vi "LIN_Data_Fold.vi"(10 "LIN Data array":T1[](array[typedef]) {"Properties" format="%x"}, 11 "Fold Data":bool) -> (2 "LIN Data array out":T1[](array[typedef]) {"Properties" format="%x"})   [LabVIEW 2014]
uses:
  Typedef/TLibLIN.ctl
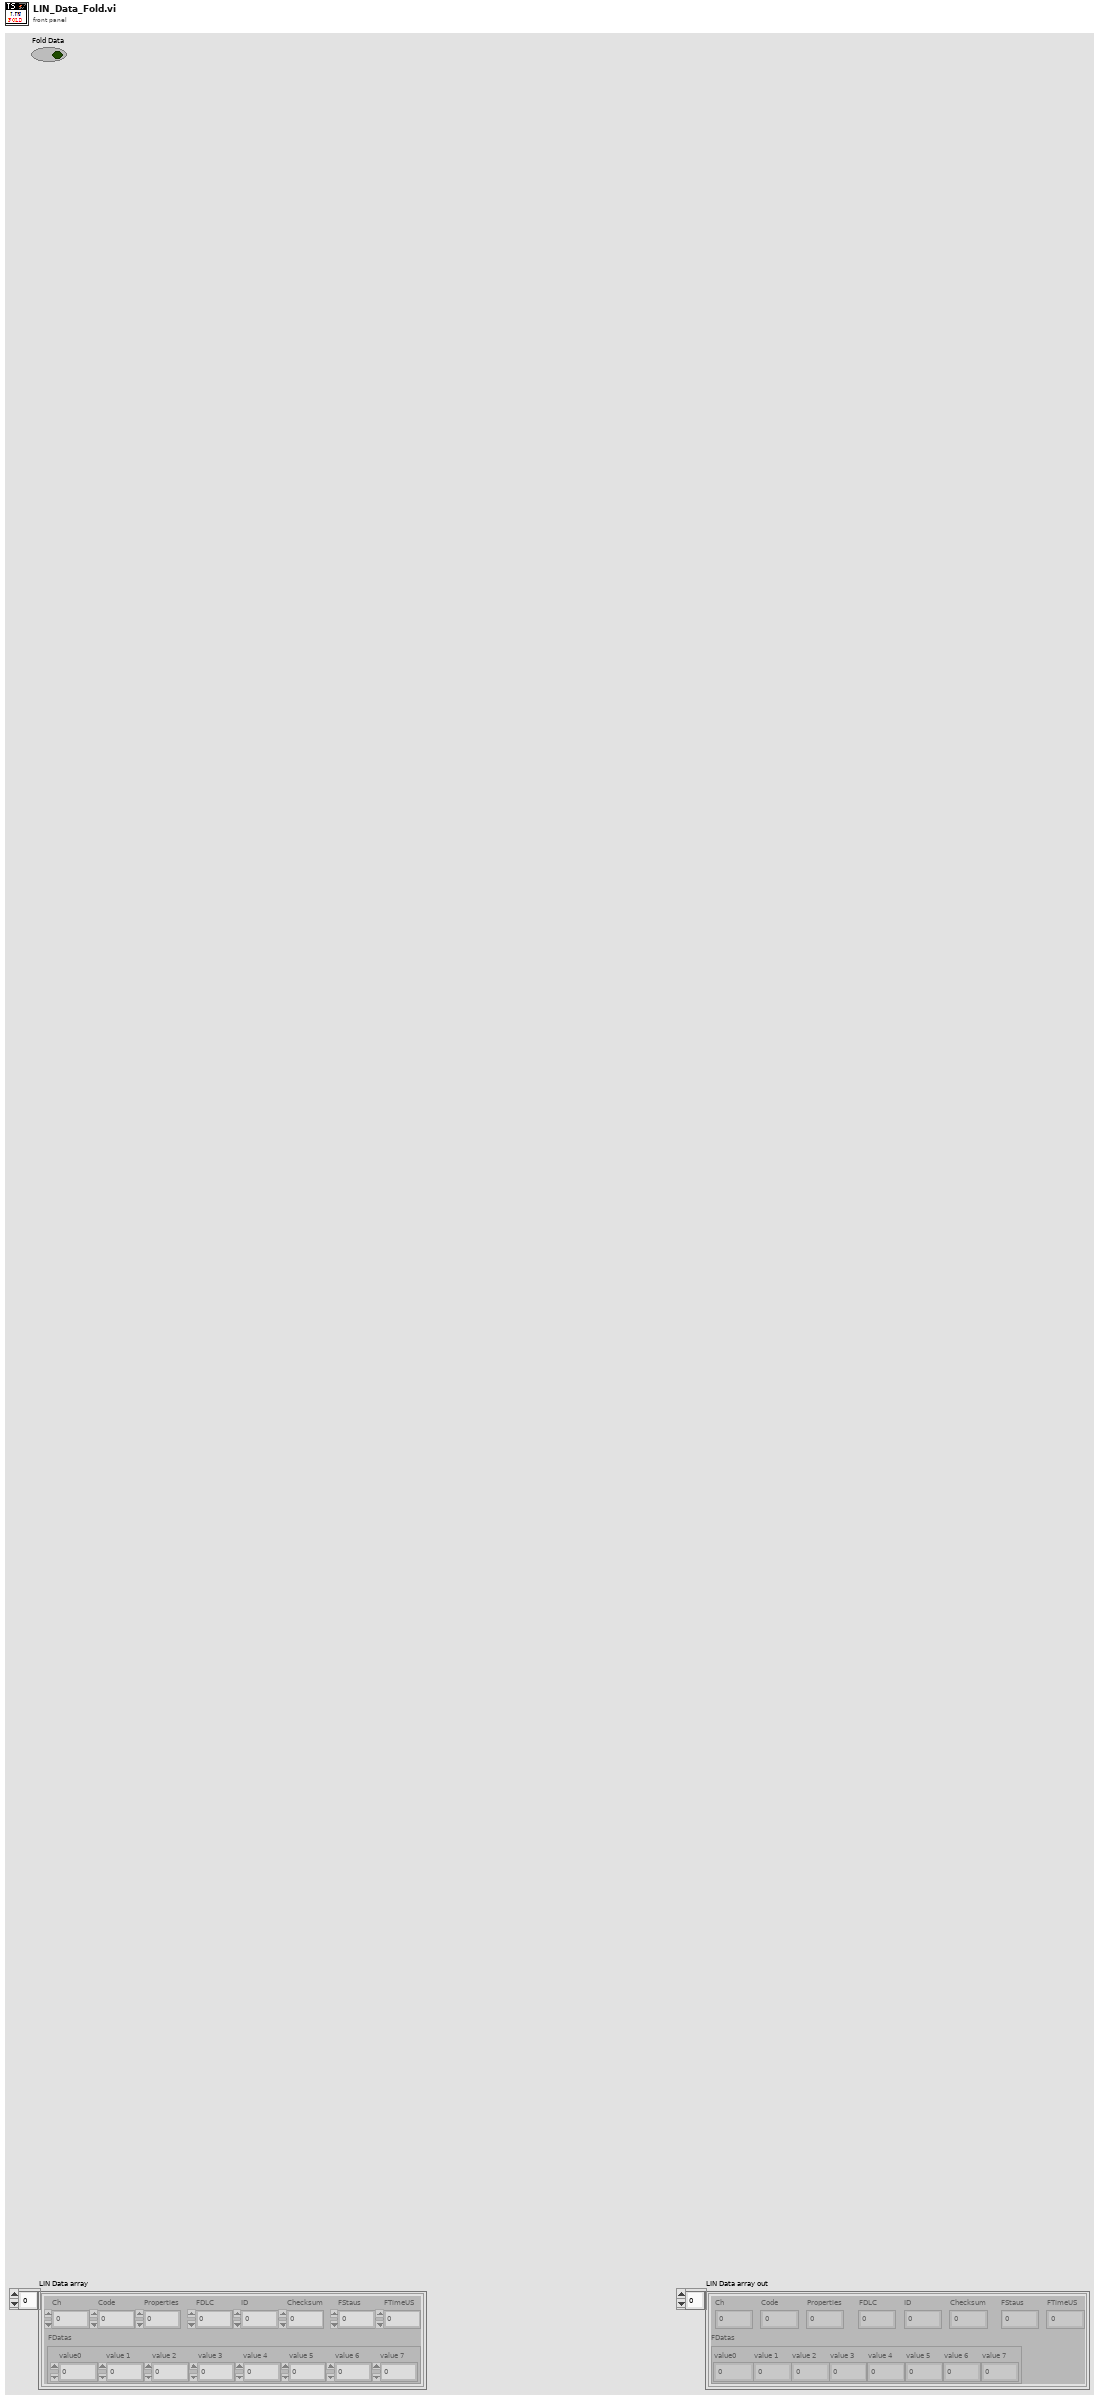
[diagram p1: front panel]
types:
  T1 = typedef "TLibLIN.ctl" = cluster{"Ch":u8, "Code":u8, "Properties":u8, "FDLC":u8, "ID":u8, "Checksum":u8, "FStaus":u8, "FTimeUS":u64, "FDatas":cluster{"value0":u8, "value 1":u8, "value 2":u8, "value 3":u8, "value 4":u8, "value 5":u8, "value 6":u8, "value 7":u8}}
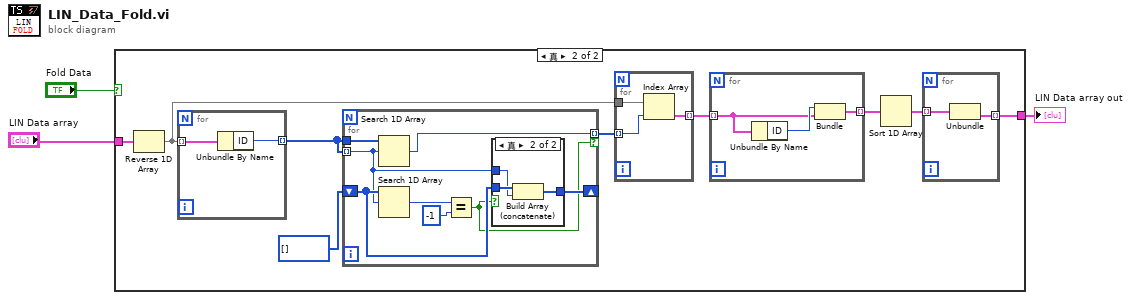
[diagram p0: block diagram]
diagram:
  n1 = case shown="真" "Fold Data" {
    tunnel: [w4 w12] -> w1
    tunnel: "LIN Data array" -> [w4 w6]
    frame False {
    }
    frame True {
      n2 = Reverse 1D Array(array=w6) -> (reversed array=w5:T1[])
      n3 = for {
        tunnel: w5 -> [w30] mode=indexing
        tunnel: [w29] -> w9 mode=indexing
        n4 = Unbundle By Name(w30) -> ("ID"=w29:u8)
      }
      n5 = for {
        tunnel: w9 -> [w19] mode=indexing
        shift-right: [w24] -> _
        shift-left: u32[] [] -> [w23]
        tunnel: [w18] -> w7 mode=indexing if=w17
        tunnel: w9 -> [w20]
        n6 = Search 1D Array(1D array=w20, element=w19) -> (index of element=w18:i32)  [unwired: 1 in]
        n7 = Search 1D Array(1D array=w23, element=w19) -> (index of element=w21:i32)  [unwired: 1 in]
        n8 = Equal?(x=w21, y=-1) -> (x = y?=w17:bool)
        n9 = case shown="真" w17 {
          tunnel: [w25 w26] -> w24
          tunnel: w23 -> [w25 w28]
          tunnel: w19 -> [_ w27]
          frame False {
          }
          frame True {
            n10 = Build Array (concatenate)(w28, w27) -> (w26:u32[])
          }
        }
      }
      n11 = for {
        tunnel: w5 -> [w16]
        tunnel: w7 -> [w15] mode=indexing
        tunnel: [w14] -> w13 mode=indexing
        n12 = Index Array(array=w16, index=w15) -> (element=w14:T1)
      }
      n13 = for {
        tunnel: w13 -> [w34] mode=indexing
        tunnel: [w33] -> w11 mode=indexing
        n14 = Unbundle By Name(w34) -> ("ID"=w35:u8)
        n15 = Bundle("ID"=w35, "ALINData"=w34) -> (w33:cluster{"ID":u8, "ALINData":T1})  [unwired: 1 in]
      }
      n16 = Sort 1D Array(array=w11) -> (sorted array=w10:cluster{"ID":u8, "ALINData":T1}[])
      n17 = for {
        tunnel: w10 -> [w32] mode=indexing
        tunnel: [w31] -> w12 mode=indexing
        n18 = Unbundle(w32) -> ("ALINData"=w31:T1)  [unwired: 1 out]
      }
    }
  }
  "LIN Data array out" <- w1
